vi "select_checked_boxes.vi"(10 "i/o array":T2(array[cluster]), 11 "checkbox array":i32[](array[numeric])) -> (0 "array of mag inputs":T1(array[cluster]), 1 "mag inputs":tag[](array[tag]), 2 "heat outputs":refnum<k21>[](array[refnum]), 3 "heat inputs":tag[](array[tag]))   [LabVIEW 2015]
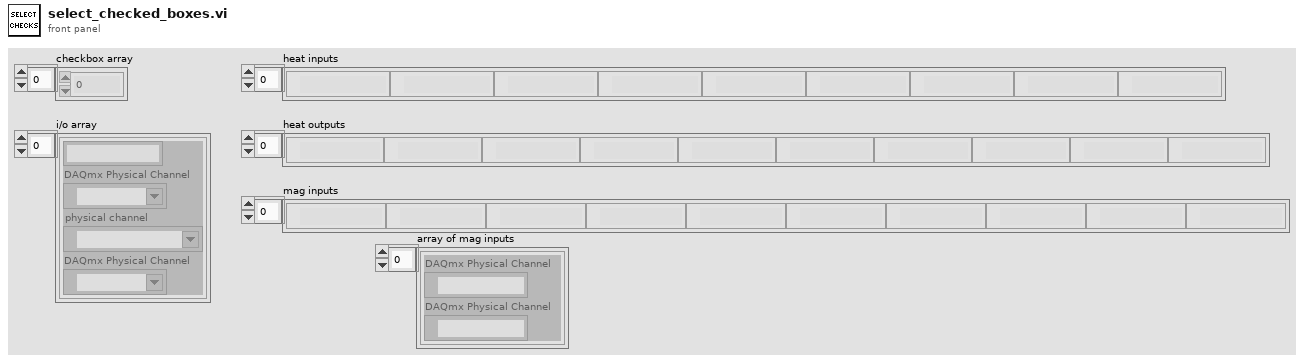
[diagram p1: front panel]
types:
  T1 = cluster{"DAQmx Physical Channel":tag, "DAQmx Physical Channel":tag}[]
  T2 = cluster{string, "DAQmx Physical Channel":tag, "physical channel":refnum<k21>, "DAQmx Physical Channel":tag}[]
  T3 = cluster{string, "DAQmx Physical Channel":tag, "physical channel":refnum<k21>, "DAQmx Physical Channel":tag}
  T4 = cluster{"DAQmx Physical Channel":tag, "DAQmx Physical Channel":tag}
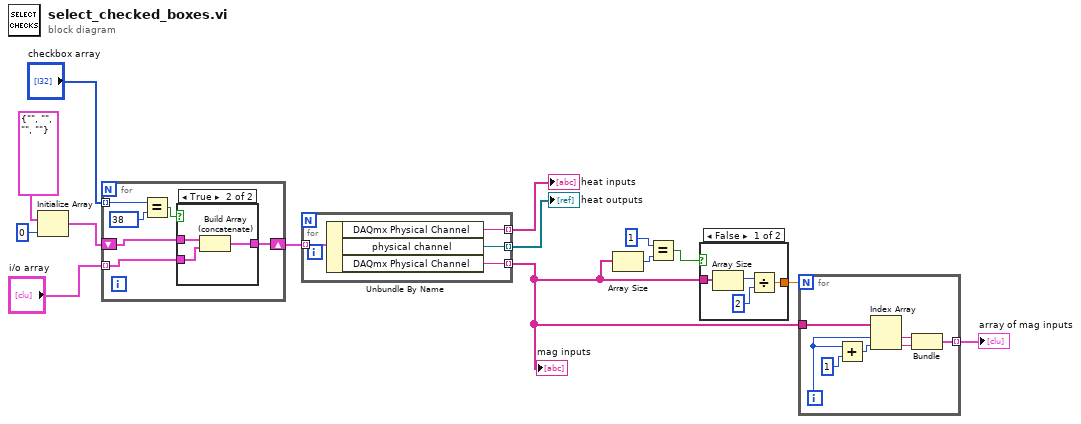
[diagram p0: block diagram]
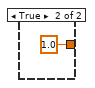
[diagram p2: hidden frame]
diagram:
  n1 = Initialize Array(T3 {"", "DAQmx Physical Channel"="", "physical channel"="", "DAQmx Physical Channel"=""} ("Cluster"), 0 ("dimension size")) -> (w12:T2)
  n2 = for {
    tunnel: "i/o array" -> [w17] mode=indexing
    tunnel: "checkbox array" -> [w19] mode=indexing
    shift-right: [w16] -> w9
    shift-left: w12 -> [w15]
    n3 = Equal?(x=w19, y=38) -> (x = y?=w18:bool)
    n4 = case shown="True" w18 {
      tunnel: w17 -> [_ w24]
      tunnel: [w21 w23] -> w16
      tunnel: w15 -> [w21 w22]
      frame False {
      }
      frame True {
        n5 = Build Array (concatenate)(w22, w24) -> (w23:T2)
      }
    }
  }
  n6 = for {
    tunnel: w9 -> [w28] mode=indexing
    tunnel: [w27] -> w13 mode=indexing
    tunnel: [w26] -> w14 mode=indexing
    tunnel: [w25] -> w4 mode=indexing
    n7 = Unbundle By Name(w28) -> ("DAQmx Physical Channel"=w27:tag, "physical channel"=w26:refnum<k21>, "DAQmx Physical Channel"=w25:tag)
  }
  "heat inputs" <- w13
  "heat outputs" <- w14
  "mag inputs" <- w4
  n8 = Array Size(array=w4) -> (size(s)=w3:i32)
  n9 = Equal?(x=1, y=w3) -> (x = y?=w1:bool)
  n10 = case shown="False" w1 {
    tunnel: [w30 1.0] -> w6
    tunnel: w4 -> [w29 _]
    frame False {
      n11 = Array Size(array=w29) -> (size(s)=w32:i32)
      n12 = Divide(x=w32, y=2) -> (x/y=w30:dbl)
    }
    frame True {
    }
  }
  n13 = for {
    N: w6 -> [_]
    tunnel: w4 -> [w40]
    tunnel: [w34] -> w5 mode=indexing
    i -> [w39]
    n14 = Add(x=w39, y=1 ("x")) -> (x+y=w37:i32)
    n15 = Index Array(array=w40, index #1=w39, index #2=w37) -> (element #1=w36:tag, element #2=w35:tag)
    n16 = Bundle("DAQmx Physical Channel"=w36, "DAQmx Physical Channel"=w35) -> (w34:T4)  [unwired: 1 in]
  }
  "array of mag inputs" <- w5
